vi "Obtain Message Queue.vi"(8 "error in (no error)":cluster{"状态":bool, "代码":i32, "源":string} caption="错误输入（无错误）") -> (0 "error out":cluster{"状态":bool, "代码":i32, "源":string} caption="错误输出", 3 "消息队列":refnum<queue>)   [LabVIEW 2014, in "Message Queue.lvlib"]
doc: "创建一个队列，数据类型为“消息簇”。"
uses:
  Message Queue.lvlib
  Message Cluster.ctl
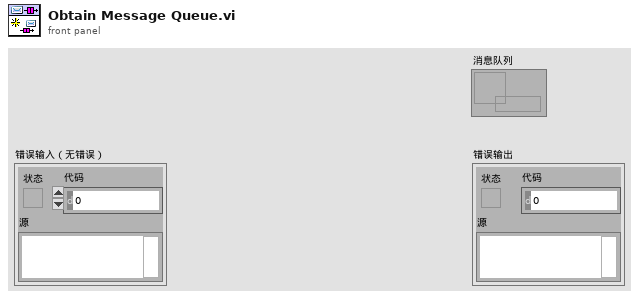
[diagram p1: front panel]
types:
  T1 = typedef "Message Queue.lvlib/Message Cluster.ctl" = cluster{"消息":string, "消息数据":variant}
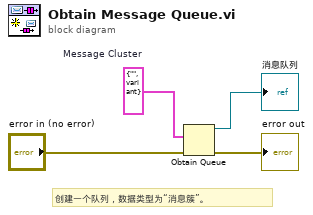
[diagram p0: block diagram]
diagram:
  w4 = T1 {"消息"="", "消息数据"=variant}  # Message Cluster
  # "创建一个队列，数据类型为“消息簇”。"
  n1 = Obtain Queue(element data type=w4, error in (no error)="error in (no error)") -> (queue out=→"消息队列":refnum<queue>, error out=→"error out":errorcluster)  [unwired: 3 in, 1 out]
